vi "File.CSV, Concatinate CSV Files In a Folder.vi"(7 "Pattern":string="*.csv", 8 "error in (no error)":errorcluster, 10 "Output Name":string="Concat CSV Files", 11 "Folder":path) -> (0 "error out":errorcluster)   [LabVIEW 2024]
uses:
  <vilib>/KATE/Files/File Utils.lvlib
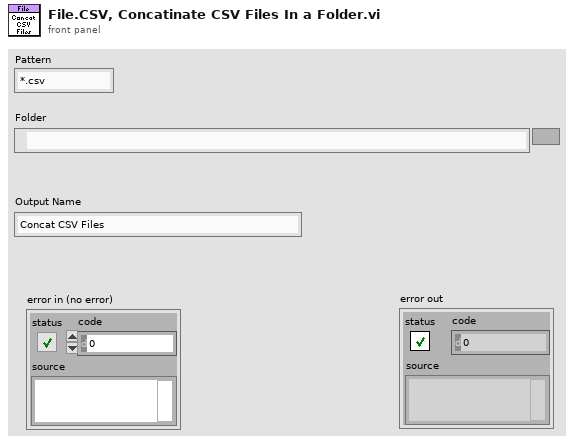
[diagram p1: front panel]
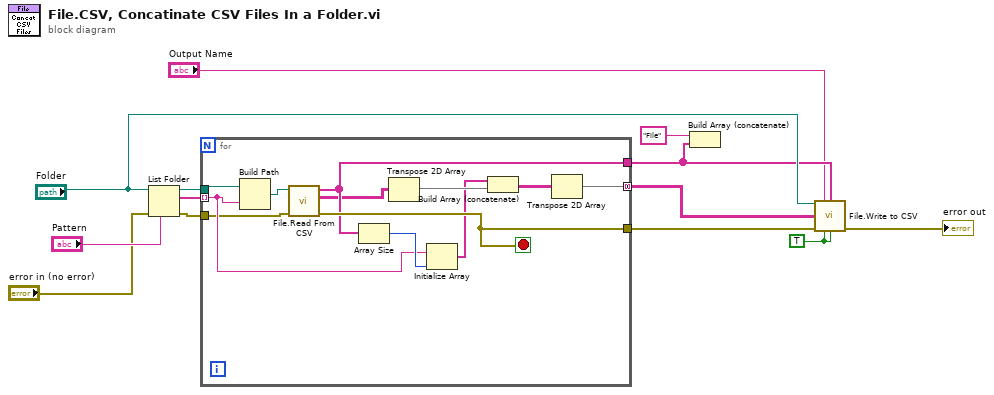
[diagram p0: block diagram]
diagram:
  w4 = TRUE ("Append Time to Filename")
  n1 = List Folder(path="Folder", pattern="Pattern", error in="error in (no error)") -> (path out=w12:path, filenames=w5:string[], error out=w1:errorcluster)  [unwired: 1 in, 1 out]
  n2 = for {
    tunnel: w12 -> [w17]
    tunnel: [w24] -> w9
    tunnel: [w25] -> w8
    tunnel: w5 -> [w16] mode=indexing
    tunnel: [w18] -> w3 mode=concatenating
    tunnel: w1 -> [w14]
    stop <- w25 stop-if-true
    n3 = Build Path(base path=w17, name or relative path=w16) -> (appended path=w15:path)
    n4 = call <vilib>:"File.Read From CSV.vi"("error in"=w14, "File"=w15) -> ("error out"=w25:errorcluster, "Data"=w22:string[][], "Header"=w24:string[])  [unwired: 7 in]
    n5 = Array Size(array=w24) -> (size(s)=w23:i32)
    n6 = Transpose 2D Array(2D array=w22) -> (transposed array=w21:string[][])
    n7 = Initialize Array(w16, w23) -> (w20:string[])
    n8 = Build Array (concatenate)(w20, w21) -> (w19:string[][])
    n9 = Transpose 2D Array(2D array=w19) -> (transposed array=w18:string[][])
  }
  n10 = Build Array (concatenate)("File", w9) -> ()  [unwired: 1 out]
  n11 = call <vilib>:"File.Write to CSV.vi"("Folder"="Folder", "FileRootName"="Output Name", "Header"=w9, "2D"=w3, "error in"=w8, "Append Time to Filename"=w4, "Append Date to Filename"=w4) -> ("error out"=→"error out":errorcluster)  [unwired: 7 in, 1 out]
